vi "两个独立循环.vi"() -> ()   [LabVIEW 2022 SP3]
doc: "本VI是为《我和LabVIEW》一书编写的示例。\n关于本书的介绍请参考网页：\nhttp://ruanqizhen.spaces.live.com/blog/cns!5852D4F797C53FB6!4310.entry"
panel:
  in  "停止":bool
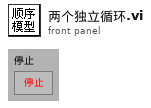
[diagram p1: front panel]
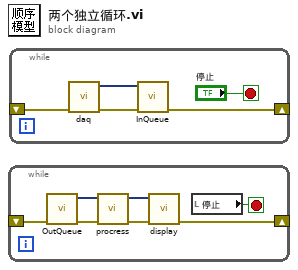
[diagram p0: block diagram]
diagram:
  n1 = while {
    shift-right: [w2] -> _
    shift-left: _ -> [w3]
    stop <- w1 stop-if-true
    n2 = call "OutQueue.vi"("error in (no error)"=w3) -> ("error out"=w4:errorcluster, "Waveform Graph"=w5:dynamicdata)  [unwired: 9 out]
    n3 = call "procress.vi"("error in (no error)"=w4, "Waveform Graph 2"=w5) -> ("error out"=w6:errorcluster, "Waveform Graph"=w7:dynamicdata)  [unwired: 8 out]
    n4 = call "display.vi"("error in (no error)"=w6, "Waveform Graph 2"=w7) -> ("error out"=w2:errorcluster)  [unwired: 9 out]
    n5 = local read "停止"() -> (w1:bool)
  }
  n6 = while {
    shift-right: [w9] -> _
    shift-left: _ -> [w12]
    stop <- "停止" stop-if-true
    n7 = call "daq.vi"("error in (no error)"=w12) -> ("error out"=w10:errorcluster, "Waveform Graph"=w11:dynamicdata)  [unwired: 9 out]
    n8 = call "InQueue.vi"("error in (no error)"=w10, "Waveform Graph 2"=w11) -> ("error out"=w9:errorcluster)  [unwired: 9 out]
  }
